vi "Practica 6 - Logaritmicos.vi"() -> ()   [LabVIEW 2023]
uses:
  <vilib>/express/express arith-compare/Formula/XNode/ExpressFormulaBlockNode.xnode
panel:
  out "Resultado Func. regulares":dbl
  out "Resultado Formula":dbl
  out "Resultado Nodo":dbl
  in  "X1":dbl
  # "Ecuacion Logaritmica"
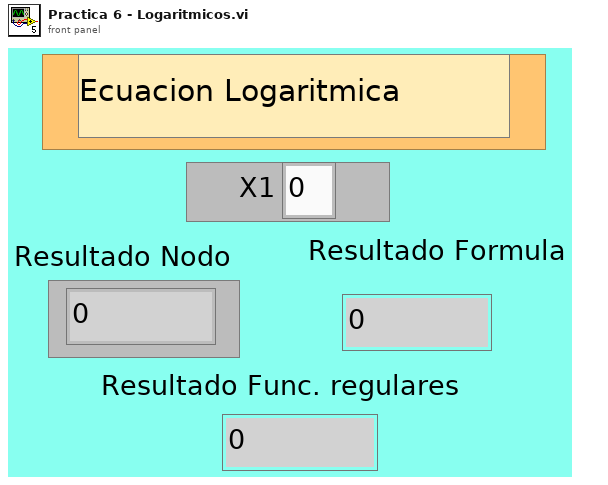
[diagram p1: front panel]
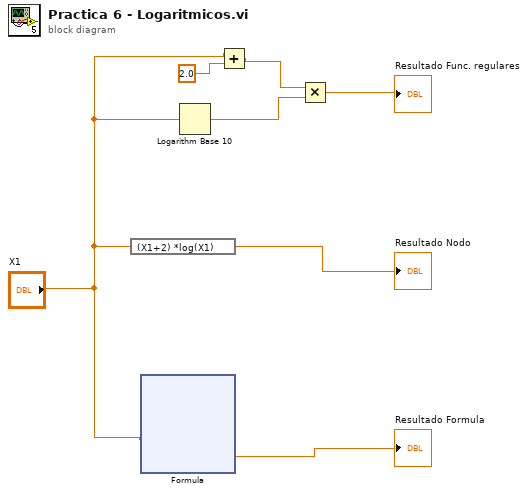
[diagram p0: block diagram]
diagram:
  n1 = expression code="(X1+2) *log(X1)"("X1") -> (→"Resultado Nodo":dbl)
  n2 = xnode "Formula"("X1"="X1") -> ("Result"=→"Resultado Formula":dbl)  [unwired: 1 in, 1 out]
  n3 = Logarithm Base 10(1:"X1") -> (0:w2:dbl)
  n4 = Add(x="X1", y=2.0) -> (x+y=w4:dbl)
  n5 = Multiply(x=w4, y=w2) -> (x*y=→"Resultado Func. regulares":dbl)
